vi "Copy Builds To NIVS Dir.vi"(5 "Files Generated by Build":path[](array[path]), 6 "Top Level/Always Included VIs":path[](array[path]), 7 "Destination Path":path, 8 "error in (no error)":errorcluster, 9 "Target Name":string, 10 "Build Specification Name":string, 11 "Project Path":path) -> (0 "error out":errorcluster)   [LabVIEW 2015]
uses:
  <vilib>/Utility/sysdir.llb/System Directory Type.ctl
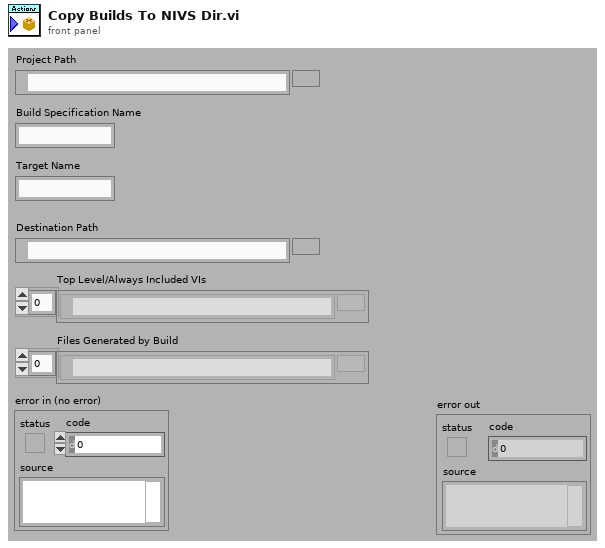
[diagram p1: front panel]
types:
  T1 = typedef "System Directory Type.ctl" = i32
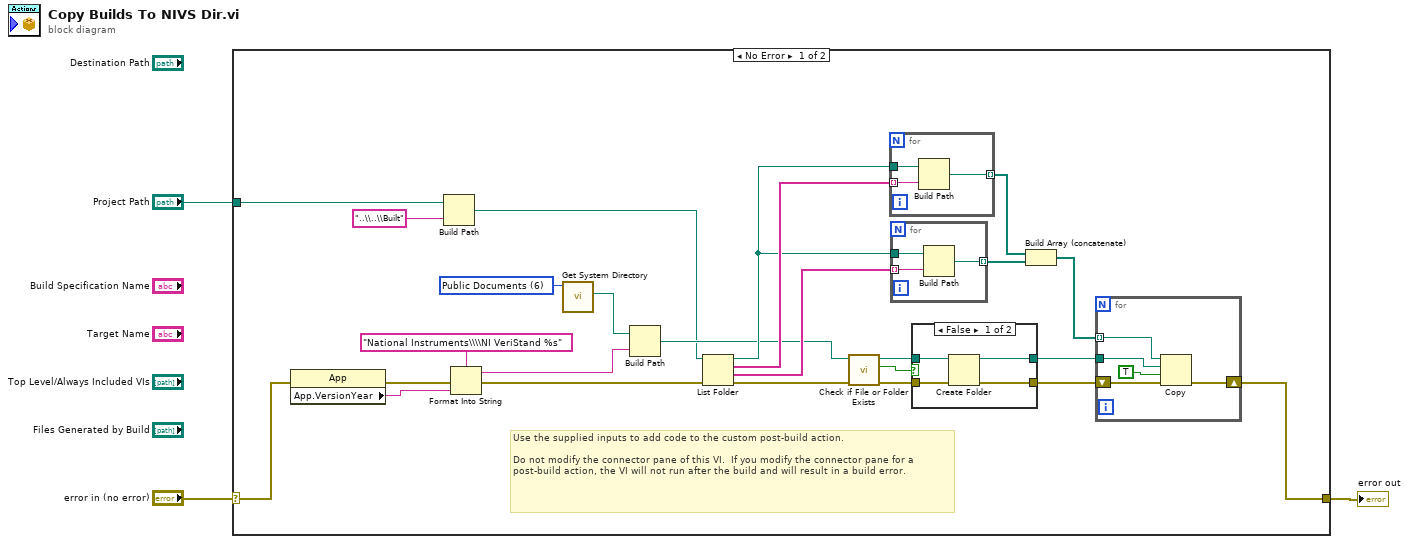
[diagram p0: block diagram]
diagram:
  n1 = case shown="No Error" "error in (no error)" {
    selector: "error in (no error)" -> [w10 w46]
    tunnel: [w12 w46] -> w1
    tunnel: "Project Path" -> [w7 _]
    frame No Error {
      w16 = T1 6 items=["User Home"=0, "User Desktop"=1, "User Documents"=2, "User Application Data"=3, "User Preferences"=4, "User Temporary"=5, "Public Documents"=6, "Public Application Data"=7, "Public Preferences"=8, "Public Cache"=13, "System Core Libraries"=9, "System Installed Libraries"=10, "Application Files"=11, "Boot Volume Root"=12] ("system directory type")
      # "Use the supplied inputs to add code to the custom post-build action.\n\nDo not modify the connector pane of this VI.  If you modify the connector pane for a post-build action, the VI will not run after the build and will result in a build error."
      n2 = property class="App"(error in=w10) -> (error out=w15:errorcluster, "App.VersionYear"=w14:string)  [unwired: 1 in, 1 out]
      n3 = Build Path(base path=w7, name or relative path="..\\..\\Built") -> (appended path=w4:path)
      n4 = Format Into String(format string="National Instruments\\\\NI VeriStand %s" ("name or relative path"), error in=w15, w14) -> (resulting string=w18:string, error out=w9:errorcluster)  [unwired: 1 in]
      n5 = call <vilib>:"Get System Directory.vi"("system directory type"=w16) -> ("system directory"=w17:path)  [unwired: 10 in]
      n6 = Build Path(base path=w17, name or relative path=w18) -> (appended path=w11:path)
      n7 = List Folder(path=w4, error in=w9) -> (path out=w21:path, filenames=w28:string[], folder names=w22:string[], error out=w19:errorcluster)  [unwired: 2 in]
      n8 = call <vilib>:"Check if File or Folder Exists.vi"("error in (no error)"=w19, "path"=w11) -> ("error out"=w23:errorcluster, "file or folder exists?"=w25:bool, "dup path"=w24:path)  [unwired: 7 in]
      n9 = for {
        tunnel: w28 -> [w44] mode=indexing
        tunnel: w21 -> [w45]
        tunnel: [w43] -> w27 mode=indexing
        n10 = Build Path(base path=w45, name or relative path=w44) -> (appended path=w43:path)
      }
      n11 = for {
        tunnel: w22 -> [w41] mode=indexing
        tunnel: w21 -> [w42]
        tunnel: [w40] -> w20 mode=indexing
        n12 = Build Path(base path=w42, name or relative path=w41) -> (appended path=w40:path)
      }
      n13 = case shown="False" w25 {
        tunnel: w24 -> [w32 w34]
        tunnel: w23 -> [w31 w33]
        tunnel: [w30 w34] -> w6
        tunnel: [w29 w33] -> w5
        frame False {
          n14 = Create Folder(path (use dialog)=w32, error in=w31) -> (created path=w30:path, error out=w29:errorcluster)  [unwired: 1 in, 1 out]
        }
        frame True {
        }
      }
      n15 = Build Array (concatenate)(w27, w20) -> (w26:path[])
      n16 = for {
        tunnel: w26 -> [w36] mode=indexing
        shift-right: [w37] -> w12
        shift-left: w5 -> [w38]
        tunnel: w6 -> [w35]
        n17 = Copy(8:w38, 9:TRUE ("overwrite (F)"), 10:w35, 11:w36) -> (0:w37:errorcluster)  [unwired: 1 in, 2 out]
      }
    }
    frame Error {
    }
  }
  "error out" <- w1
